vi "PH_Calorimeter_USB.ProcEvents.vi"(0 "i ref in":refnum<vi>, 5 "error in":errorcluster) -> (14 "i ref out":refnum<vi>, 19 "error out":errorcluster)   [LabVIEW 2014, in "PH_Calorimeter_USB.lvlib"]
doc: "This method is used to define the events the object will listen to. Add your own events here."
uses:
  PH_Calorimeter_USB.lvlib
  CS_Core/BaseProcess/BaseProcess.event definition.ctl
  CS_Core/CAEObj/CAEObj.event definition.ctl
  CS_Core/BaseProcess/BaseProcess.descriptor string definition.ctl
  CS_Core/BaseProcess/BaseProcess.lvlib
  CS_Core/CAEObj/CAEObj.lvlib
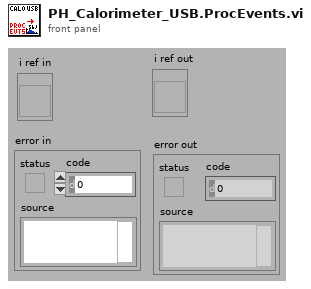
[diagram p1: front panel]
types:
  T1 = typedef "BaseProcess.lvlib/BaseProcess.event definition.ctl" = cluster{"CAEEvtDef":T2, "Data Descriptor":T3}
  T2 = typedef "CAEObj.lvlib/CAEObj.event definition.ctl" = cluster{"URL":string, "enable":bool, "ignoreResID":bool}
  T3 = typedef "BaseProcess.lvlib/BaseProcess.descriptor string definition.ctl" = string
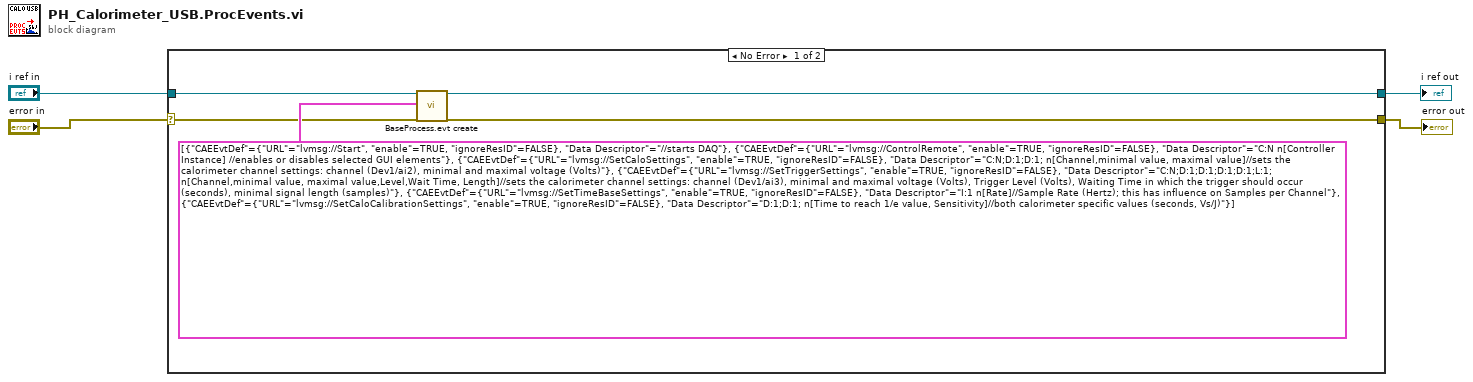
[diagram p0: block diagram]
diagram:
  n1 = case shown="No Error" "error in" {
    selector: "error in" -> [w5 w10]
    tunnel: "i ref in" -> [w9 w11]
    tunnel: [w7 w10] -> w3
    tunnel: [w6 w11] -> w2
    frame No Error {
      n2 = call "BaseProcess.evt create.vi"("i ref in"=w9, "newEvents"=T1[] [{"CAEEvtDef"={"URL"="lvmsg://Start", "enable"=TRUE, "ignoreResID"=FALSE}, "Data Descriptor"="//starts DAQ"}, {"CAEEvtDef"={"URL"="lvmsg://ControlRemote", "enable"=TRUE, "ignoreResID"=FALSE}, "Data Descriptor"="C:N n[Controller Instance] //enables or disables selected GUI elements"}, {"CAEEvtDef"={"URL"="lvmsg://SetCaloSettings", "enable"=TRUE, "ignoreResID"=FALSE}, "Data Descriptor"="C:N;D:1;D:1; n[Channel,minimal value, maximal value]//sets the calorimeter channel settings: channel (Dev1/ai2), minimal and maximal voltage (Volts)"}, {"CAEEvtDef"={"URL"="lvmsg://SetTriggerSettings", "enable"=TRUE, "ignoreResID"=FALSE}, "Data Descriptor"="C:N;D:1;D:1;D:1;D:1;L:1; n[Channel,minimal value, maximal value,Level,Wait Time, Length]//sets the calorimeter channel settings: channel (Dev1/ai3), minimal and maximal voltage (Volts), Trigger Level (Volts), Waiting Time in which the trigger should occur (seconds), minimal signal length (samples)"}, {"CAEEvtDef"={"URL"="lvmsg://SetTimeBaseSettings", "enable"=TRUE, "ignoreResID"=FALSE}, "Data Descriptor"="I:1 n[Rate]//Sample Rate (Hertz); this has influence on Samples per Channel"}, {"CAEEvtDef"={"URL"="lvmsg://SetCaloCalibrationSettings", "enable"=TRUE, "ignoreResID"=FALSE}, "Data Descriptor"="D:1;D:1; n[Time to reach 1/e value, Sensitivity]//both calorimeter specific values (seconds, Vs/J)"}] ("new events"), "error in (no error)"=w5) -> ("i ref out"=w6:refnum<vi>, "error out"=w7:errorcluster)  [unwired: 13 in, 2 out]
    }
    frame Error {
    }
  }
  "i ref out" <- w2
  "error out" <- w3
